vi "LoadControlPanel.vi"(8 "error in (no error)":errorcluster, 10 "Actor In":refnum<class "Actor.lvclass">, 11 "GRMActor in":refnum<class "Displayer.lvclass">) -> (0 "error out":errorcluster, 3 "GRMActor out":refnum<class "Displayer.lvclass">)   [LabVIEW 2020, in "Displayer.lvlib" / "Displayer.lvclass"]
uses:
  Displayer.lvclass
  <vilib>/ActorFramework/Actor/Actor.lvclass
  DisplayerUI/DisplayerUI.lvclass
  C:/Program Files/National Instruments/LabVIEW 2020/vi.lib/ActorFramework/Actor/Actor.lvclass
  Model/Hardware Abstraction Layer/Component/Device/Device/DataExchange.ctl
  Model/Hardware Abstraction Layer/Component/GenericActor/GenericActor/GenericActor.lvclass
  Interface/DataListener/DataListener.lvclass
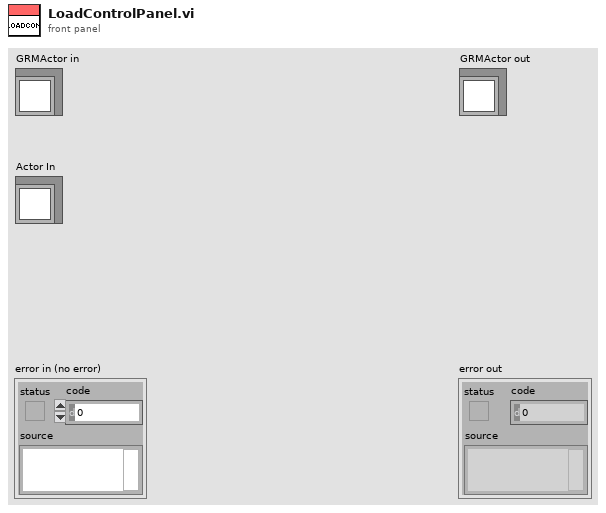
[diagram p1: front panel]
types:
  T1 = typedef "DataListener.lvclass/DataExchange.ctl" = cluster{"Source":string, "Destination":string, "Description":string, "value":variant}
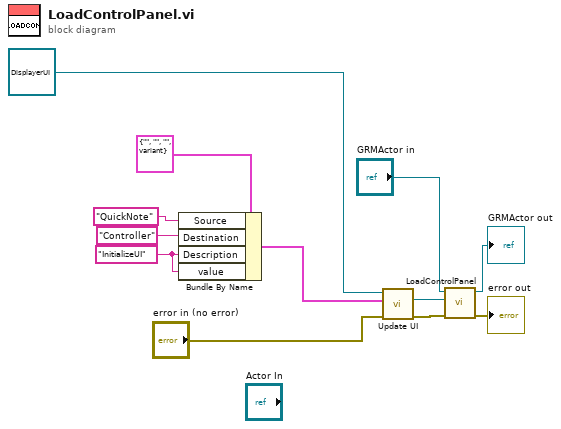
[diagram p0: block diagram]
diagram:
  w5 = "InitializeUI" ("Description")
  n1 = Bundle By Name(cluster=T1 {"Source"="", "Destination"="", "Description"="", "value"=variant} ("DataExchange"), "Source"="QuickNote", "Destination"="Controller", "Description"=w5, "value"=w5) -> (w1:T1)
  n2 = call-dynamic "Update UI.vi"("error in (no error)"="error in (no error)", "DataExchange"=w1, "Controller Template in"=refnum<class "DisplayerUI.lvclass"> refnum ("Displayer.lvlib:DisplayerUI.lvlib:DisplayerUI.lvclass")) -> ("error out"=w4:errorcluster, "Controller Template out"=w2:refnum<class "DisplayerUI.lvclass">)  [unwired: 7 in]
  n3 = call-parent "LoadControlPanel.vi"("error in (no error)"=w4, "Actor In"=w2, "GRMActor in"="GRMActor in") -> ("error out"=→"error out":errorcluster, "GRMActor out"=→"GRMActor out":refnum<class "Displayer.lvclass">)  [unwired: 7 in]
